vi "drive train pid.vi"(0 "Boolean":bool, 2 "leftDrive":dbl, 3 "rightDrive":dbl, 5 "Cluster":T1, 6 "leftReqVel":dbl, 7 "rightReqVel":dbl, 8 "rightVelocity":dbl, 9 "leftVelocity":dbl) -> (14 "Left Motor Power out":dbl, 19 "Right Motor Power out":dbl)   [LabVIEW 2013]
uses:
  Drive Train Metrics.ctl
  CmdFlag.ctl
  <vilib>/addons/control/pid/pid.llb/PID (DBL).vi
  <vilib>/addons/control/pid/NI_PID_pid.lvlib
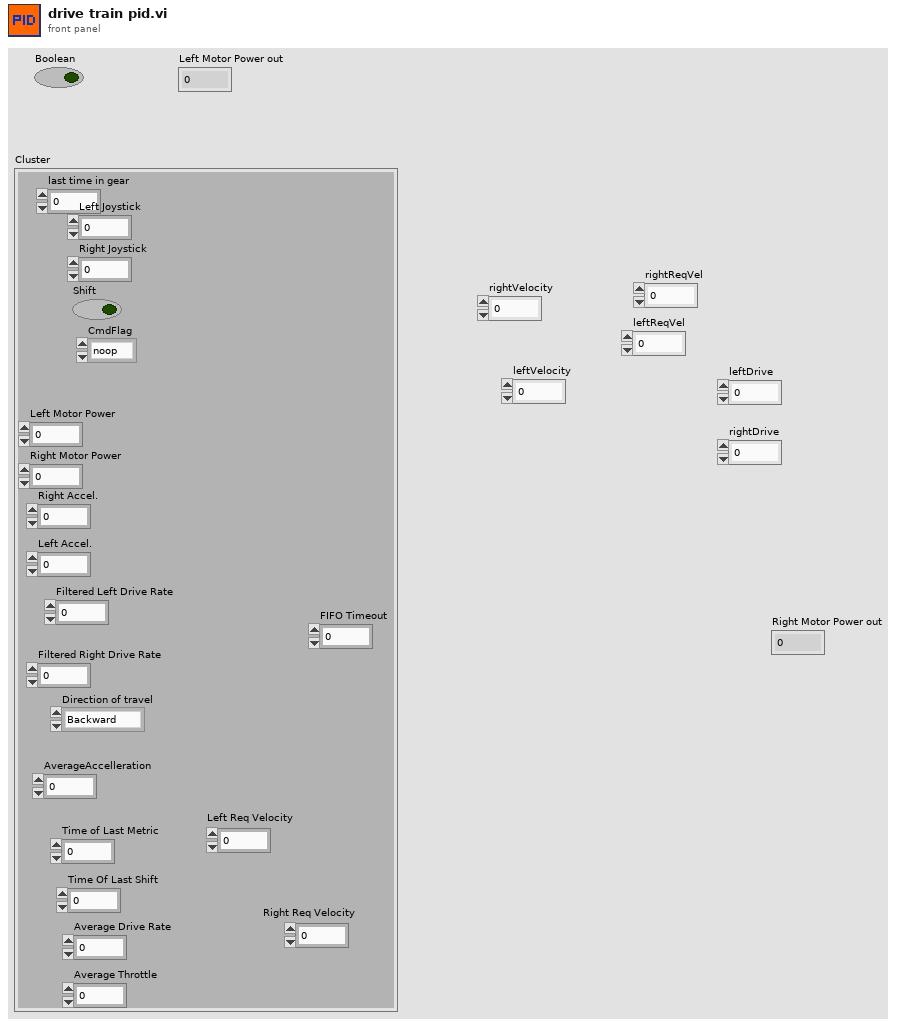
[diagram p1: front panel]
types:
  T1 = typedef "Drive Train Metrics.ctl" = cluster{"last time in gear":u32, "Shift":bool, "Right Joystick":dbl, "Left Joystick":dbl, "CmdFlag":T2, "Right Motor Power":dbl, "Left Motor Power":dbl, "Right Accel.":dbl, "Left Accel.":dbl, "Filtered Left Drive Rate":dbl, "Filtered Right Drive Rate":dbl, "Direction of travel":enum16{"Backward", "Forward", "Spin"}, "AverageAccelleration":dbl, "Time of Last Metric":u32, "Time Of Last Shift":dbl, "Average Drive Rate":dbl, "Average Throttle":dbl, "FIFO Timeout":i32, "Left Req Velocity":dbl, "Right Req Velocity":dbl}
  T2 = typedef "CmdFlag.ctl" = enum16{"noop", "suspend", "resume"}
  T3 = cluster{"proportional gain (Kc)":dbl, "integral time (Ti, min)":dbl, "derivative time (Td, min)":dbl}
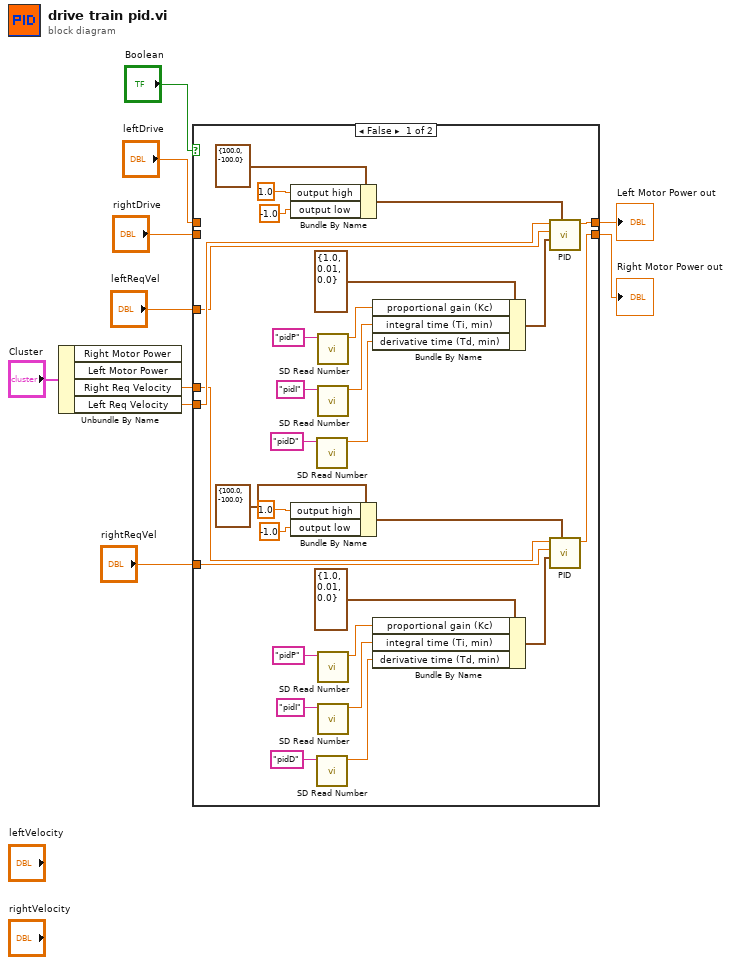
[diagram p0: block diagram]
diagram:
  n1 = Unbundle By Name("Cluster") -> ("Right Req Velocity"=w7:dbl, "Left Req Velocity"=w8:dbl)  [unwired: 2 out]
  n2 = case shown="False" "Boolean" {
    tunnel: [w38 w41] -> w6
    tunnel: w8 -> [w27 _]
    tunnel: w7 -> [w14 _]
    tunnel: [w13 w42] -> w5
    tunnel: "leftReqVel" -> [w12 _]
    tunnel: "rightReqVel" -> [w11 _]
    tunnel: "rightDrive" -> [_ w42]
    tunnel: "leftDrive" -> [_ w41]
    frame False {
      n3 = Bundle By Name(cluster=cluster{"output high":dbl, "output low":dbl} {"output high"=100.0, "output low"=-100.0} ("output range"), "output high"=1.0, "output low"=-1.0) -> (w36:cluster{"output high":dbl, "output low":dbl})
      n4 = Bundle By Name(cluster=cluster{"output high":dbl, "output low":dbl} {"output high"=100.0, "output low"=-100.0} ("output range"), "output high"=1.0, "output low"=-1.0) -> (w15:cluster{"output high":dbl, "output low":dbl})
      n5 = call <vilib>:"SD Read Number.vi"("Name"="pidD") -> ("Numeric"=w28:dbl)  [unwired: 8 in, 2 out]
      n6 = call <vilib>:"SD Read Number.vi"("Name"="pidD") -> ("Numeric"=w17:dbl)  [unwired: 8 in, 2 out]
      n7 = call <vilib>:"SD Read Number.vi"("Name"="pidP") -> ("Numeric"=w32:dbl)  [unwired: 8 in, 2 out]
      n8 = call <vilib>:"SD Read Number.vi"("Name"="pidI") -> ("Numeric"=w29:dbl)  [unwired: 8 in, 2 out]
      n9 = call <vilib>:"SD Read Number.vi"("Name"="pidP") -> ("Numeric"=w21:dbl)  [unwired: 8 in, 2 out]
      n10 = call <vilib>:"SD Read Number.vi"("Name"="pidI") -> ("Numeric"=w18:dbl)  [unwired: 8 in, 2 out]
      n11 = Bundle By Name(cluster=T3 {"proportional gain (Kc)"=1.0, "integral time (Ti, min)"=0.01, "derivative time (Td, min)"=0.0} ("PID gains"), "proportional gain (Kc)"=w32, "integral time (Ti, min)"=w29, "derivative time (Td, min)"=w28) -> (w39:T3)
      n12 = Bundle By Name(cluster=T3 {"proportional gain (Kc)"=1.0, "integral time (Ti, min)"=0.01, "derivative time (Td, min)"=0.0} ("PID gains"), "proportional gain (Kc)"=w21, "integral time (Ti, min)"=w18, "derivative time (Td, min)"=w17) -> (w25:T3)
      n13 = call-poly <vilib>:"PID.vi"("output range"=w36, "PID gains"=w39, "process variable"=w12, "setpoint"=w27) -> ("output"=w38:dbl)  [unwired: 6 in, 1 out]
      n14 = call-poly <vilib>:"PID.vi"("output range"=w15, "PID gains"=w25, "process variable"=w11, "setpoint"=w14) -> ("output"=w13:dbl)  [unwired: 6 in, 1 out]
    }
    frame True {
    }
  }
  "Left Motor Power out" <- w6
  "Right Motor Power out" <- w5
